vi "Insight_Telnet_Test.vi"() -> ()   [LabVIEW 2011]
panel:
  in  "remote port (23)":u16=23
  in  "stop":bool
  out "error out":errorcluster
  in  "error in (no error)":errorcluster
  in  "IP Address":string="192.168.1.151"
  in  "Method":enum16{"Telnet Open", "Telnet Close"}(ring)
  out "response data":string
  in  "Timeout, sec":u32=3
  in  "write buffer (\"\")":string
  in  "Send Command":bool
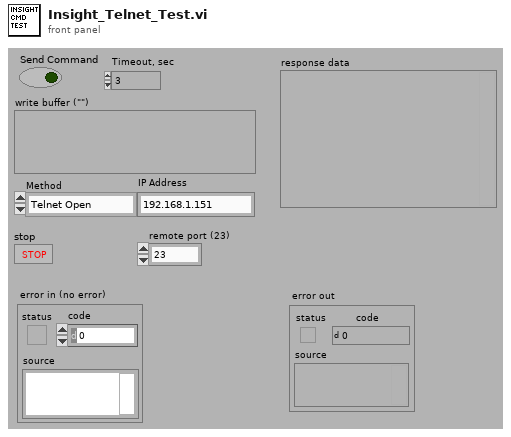
[diagram p1: front panel]
types:
  T1 = typedef "Telnet Session.ctl" = refnum<k1>
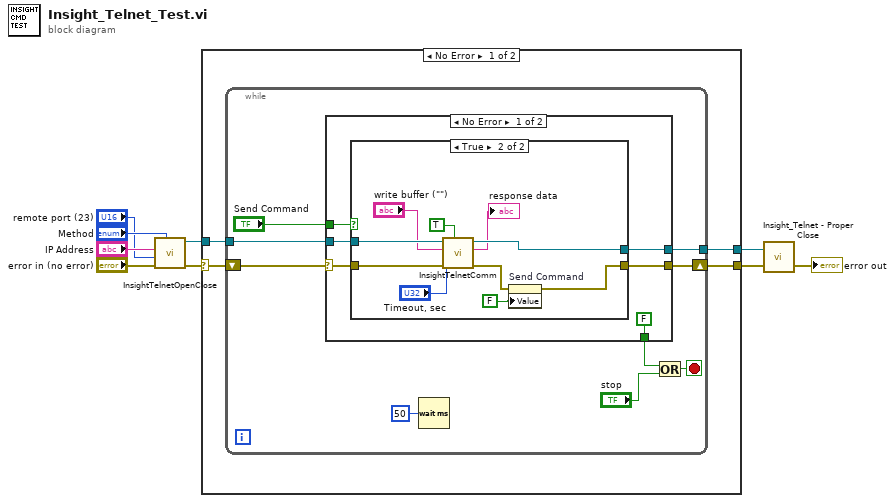
[diagram p0: block diagram]
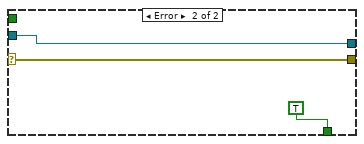
[diagram p3: hidden frame]
diagram:
  n1 = call "InsightTelnetOpenClose.vi"("IP Address"="IP Address", "remote port (23)"="remote port (23)", "error in (no error)"="error in (no error)", "Method"="Method") -> ("telnet connection"=w7:T1, "error out"=w9:errorcluster)  [unwired: 5 in]
  n2 = case shown="No Error" w9 {
    selector: w9 -> [w10 w45]
    tunnel: [w11 w45] -> w8
    tunnel: w7 -> [w13 w44]
    tunnel: [w12 w44] -> w6
    frame No Error {
      n3 = while {
        tunnel: w13 -> [w20]
        tunnel: [w19] -> w12
        shift-right: [w18] -> w11
        shift-left: w10 -> [w17]
        stop <- w14 stop-if-true
        n4 = case shown="No Error" w17 {
          selector: w17 -> [w24 w43]
          tunnel: "Send Command" -> [w28 _]
          tunnel: w20 -> [w27 w42]
          tunnel: [w26 w42] -> w19
          tunnel: [w25 w43] -> w18
          tunnel: [FALSE TRUE] -> w16
          frame No Error {
            n5 = case shown="True" w28 {
              tunnel: w24 -> [w30 w40]
              tunnel: [w30 w32] -> w25
              tunnel: w27 -> [w29 w39]
              tunnel: [w29 w38] -> w26
              frame False {
              }
              frame True {
                n6 = call "InsightTelnetComm.vi"("Continue on 6002 Error (FALSE)"=TRUE, "error in"=w40, "Timeout, sec"="Timeout, sec", "write buffer (\"\")"="write buffer (\"\")", "telnet connection"=w39) -> ("error out"=w33:errorcluster, "response data"=→"response data":string, "telnet  connection out"=w38:T1)  [unwired: 2 in]
                n7 = property on="Send Command" class="Bool (strict)"(error in=w33, "Value"=FALSE ("Send Command")) -> (error out=w32:errorcluster)  [unwired: 1 in, 1 out]
              }
            }
          }
          frame Error {
          }
        }
        n8 = Wait (ms)(milliseconds to wait=u32 50) -> ()  [unwired: 1 out]
        n9 = Or(x=w16, y="stop") -> (x .or. y?=w14:bool)
      }
    }
    frame Error {
    }
  }
  n10 = call "Insight_Telnet - Proper Close.vi"("error in"=w8, "telnet connection"=w6) -> ("error out"=→"error out":errorcluster)  [unwired: 1 in]
